vi "Perform Measurement - Single Point.vi"(8 "error in (no error)":errorcluster, 9 "Measure Call Context in":refnum<class "Measure Call Context.lvclass">, 11 "measurement configuration":T2={"Mode of operation"=enum."Power on the DUT", "Source enable/disable"=FALSE, "Load enable/disable"=FALSE, "Power ON/Source resource names"=[], "Load resource names"=[], "Power ON/Source system configuration"=enum."Series", "Power ON/Source output function"=0, "Power ON/Source voltage/current level"=0.0, "Source voltage/current level range"=0.0, "Power ON/Source sense"=0, "Source limit symmetry"=enum."Symmetric", "Power ON/Source current/voltage limit range"=0.0, "Source current/voltage limit low"=0.0, "Source current/voltage limit high"=0.0, "Source transient response"=0, "Source voltage gain bandwidth"=0.0, "Source voltage compensation frequency"=0.0, "Load device voltage/current rating"=30.0, "Source voltage pole-zero ratio"=0.0, "Load system configuration"=enum."Series", "Load output function"=0, "Load voltage/current level"=0.0, "Load voltage/current level range"=0.0, "Load sense"=0, "Load limit symmetry"=enum."Symmetric", "Load current/voltage limit range"=0.0, "Load current/voltage limit low"=0.0, "Load current/voltage limit high"=0.0, "Load transient response"=0, "Load current gain bandwidth"=0.0, "Load current compensation frequency"=0.0, "Load current pole-zero ratio"=0.0, "Aperture time"=0.0, "Measurement duration"=0.0, "Measurement timeout"=1.0} {"Measurement timeout" format="%.3p"; "Load device voltage/current rating" format="%#_6pA"; "Load current compensation frequency" format="%#_6p"; "Load output function" items=["DC Voltage"=1006, "DC Current"=1007, "Pulse Voltage"=1049, "Pulse Current"=1050]; "Power ON/Source output function" items=["DC Voltage"=1006, "DC Current"=1007, "Pulse Voltage"=1049, "Pulse Current"=1050]; "Load sense" items=["Local"=1008, "Remote"=1009]; "Load transient response" items=["Slow"=1041, "Normal"=1038, "Fast"=1039, "Custom"=1042]; "Power ON/Source sense" items=["Symmetric", "Asymmetric"]; "Source transient response" items=["Slow"=1041, "Normal"=1038, "Fast"=1039, "Custom"=1042]; "Measurement duration" format="%.3p"; "Load current/voltage limit high" format="%#_6p"; "Load current/voltage limit low" format="%#_6p"; "Load current/voltage limit range" format="%#_6p"; "Load voltage/current level range" format="%#_6p"; "Load voltage/current level" format="%#_6p"; "Source current/voltage limit high" format="%#_6p"; "Source current/voltage limit low" format="%#_6p"; "Power ON/Source current/voltage limit range" format="%#_6p"; "Source voltage/current level range" format="%#_6p"; "Power ON/Source voltage/current level" format="%#_6p"}) -> (0 "error out":errorcluster, 1 "Measure Call Context out":refnum<class "Measure Call Context.lvclass">, 3 "Measurement Results":T1)   [LabVIEW 2021, in "Single Point_Channel Ganging.lvlib"]
doc: "This VI Perform different API calls to do Single-Point Measurement in different configurations of Source and Load like \n\nSingle-Ganged \nGanged-Ganged\nGanged-Single\nSingle-Single"
uses:
  Single Point_Channel Ganging.lvlib
  Measurement Configuration.ctl
  Measurement Results.ctl
  <vilib>/Plug-In SDKs/Measurements/Measure Call Context/Measure Call Context.lvclass
  Controls/Perform measurement-control.ctl
  shared subVIs/ctl/NIDCPower_channel_ganging - ctl - ganged session.ctl
  shared subVIs/ctl/NIDCPower_channel_ganging - ctl - ganged config.ctl
  shared subVIs/ctl/NIDCPower_channel_ganging - ctl - channel mode.ctl
  <instrlib>/niDCPower/nidcpower.llb/niDCPower Wait For Event - Event.ctl
  shared/Common/controls/Start and Wait for Event.ctl
  shared/Ganging/controls/Abort Single Point-Ganging.ctl
  shared/Single/controls/Abort Single Point-Single.ctl
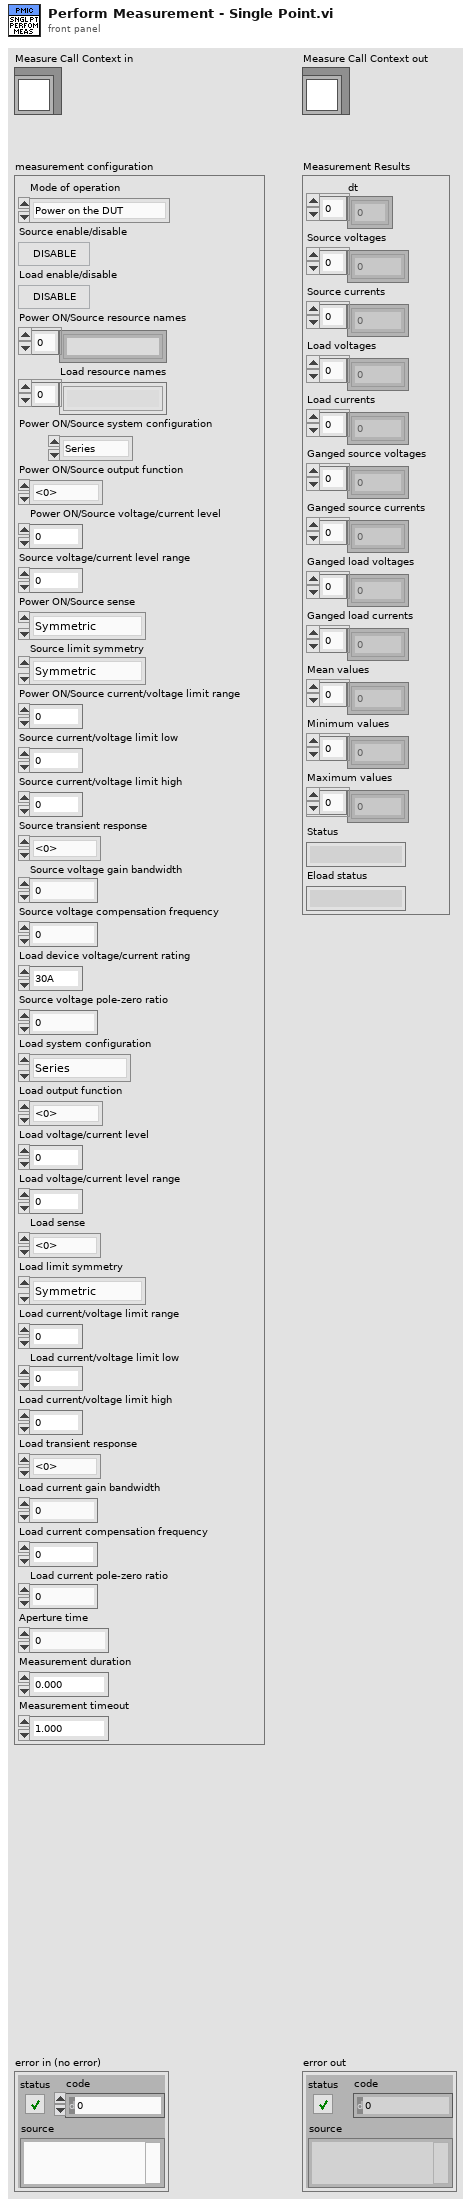
[diagram p1: front panel]
types:
  T1 = typedef "Single Point_Channel Ganging.lvlib/Measurement Results.ctl" = cluster{"dt":dbl[], "Source voltages":dbl[], "Source currents":dbl[], "Load voltages":dbl[], "Load currents":dbl[], "Ganged source voltages":dbl[], "Ganged source currents":dbl[], "Ganged load voltages":dbl[], "Ganged load currents":dbl[], "Mean values":dbl[], "Minimum values":dbl[], "Maximum values":dbl[], "Status":string, "Eload status":string}
  T2 = typedef "Single Point_Channel Ganging.lvlib/Measurement Configuration.ctl" = cluster{"Mode of operation":enum32{"Power on the DUT", "Perform measurement", "Power off the DUT"}, "Source enable/disable":bool, "Load enable/disable":bool, "Power ON/Source resource names":string[], "Load resource names":string[], "Power ON/Source system configuration":enum32{"Series", "Parallel", "Manual"}, "Power ON/Source output function":i32, "Power ON/Source voltage/current level":dbl, "Source voltage/current level range":dbl, "Power ON/Source sense":i32, "Source limit symmetry":enum32{"Symmetric", "Asymmetric"}, "Power ON/Source current/voltage limit range":dbl, "Source current/voltage limit low":dbl, "Source current/voltage limit high":dbl, "Source transient response":i32, "Source voltage gain bandwidth":dbl, "Source voltage compensation frequency":dbl, "Load device voltage/current rating":dbl, "Source voltage pole-zero ratio":dbl, "Load system configuration":enum32{"Series", "Parallel", "Manual"}, "Load output function":i32, "Load voltage/current level":dbl, "Load voltage/current level range":dbl, "Load sense":i32, "Load limit symmetry":enum32{"Symmetric", "Asymmetric"}, "Load current/voltage limit range":dbl, "Load current/voltage limit low":dbl, "Load current/voltage limit high":dbl, "Load transient response":i32, "Load current gain bandwidth":dbl, "Load current compensation frequency":dbl, "Load current pole-zero ratio":dbl, "Aperture time":dbl, "Measurement duration":dbl, "Measurement timeout":dbl}
  T3 = typedef "Single Point_Channel Ganging.lvlib/Perform measurement-control.ctl" = cluster{"Source Ganged Session Out":T4, "Load Ganged Session Out":T4, "Source Measure Record Length":i32, "Load Measure Record Length":i32, "Measurement Results":T1, "Load Slave resource name":string[], "Load Master/Single resource name":string, "Source Slave resource name":string[], "Source Master/Single resource name":string, "Load ganged/single":bool, "Source ganged/single":bool, "Source channel name":string, "Load channel name":string, "Source session out":refnum<k15>, "Load session out":refnum<k15>, "Number of Eload used":i32, "Load Source ON/OFF":enum16{"SOURCE AND LOAD OFF", "SOURCE ON", "LOAD ON", "SOURCE AND LOAD ON"}, "Measurement timeout":dbl}
  T4 = typedef "NIDCPower_channel_ganging - ctl - ganged session.ctl" = cluster{"Ganged Config":T5, "Session List":refnum<k15>[], "Session Mode":T6[], "Channel":string[]}
  T5 = typedef "NIDCPower_channel_ganging - ctl - ganged config.ctl" = enum32{"Series", "Parallel", "Manual"}
  T6 = typedef "NIDCPower_channel_ganging - ctl - channel mode.ctl" = enum32{"Master", "Slave", "Slave - Inverted"}
  T7 = typedef "Start and Wait for Event.ctl" = cluster{"Source Ganged Session Out":T4, "Load Ganged Session Out":T4, "Source session out":refnum<k15>, "Load session out":refnum<k15>, "event":T8, "Source channel name":string, "Load channel name":string, "Load Source ON/OFF":enum16{"SOURCE AND LOAD OFF", "SOURCE ON", "LOAD ON", "SOURCE AND LOAD ON"}, "Load ganged/single":bool, "Source ganged/single":bool}
  T8 = typedef "niDCPower Wait For Event - Event.ctl" = i32
  T9 = typedef "Abort Single Point-Ganging.ctl" = cluster{"Ganged Session in":cluster{"Ganged Config":T5, "Session List":refnum<k15>[], "Session Mode":T6[], "Channel":string[]}}
  T10 = typedef "Abort Single Point-Single.ctl" = cluster{"Resource out":refnum<k15>, "Resource channel name":string}
  T11 = enum32{"Power on the DUT", "Perform measurement", "Power off the DUT"}
  T12 = enum16{"SOURCE AND LOAD OFF", "SOURCE ON", "LOAD ON", "SOURCE AND LOAD ON"}
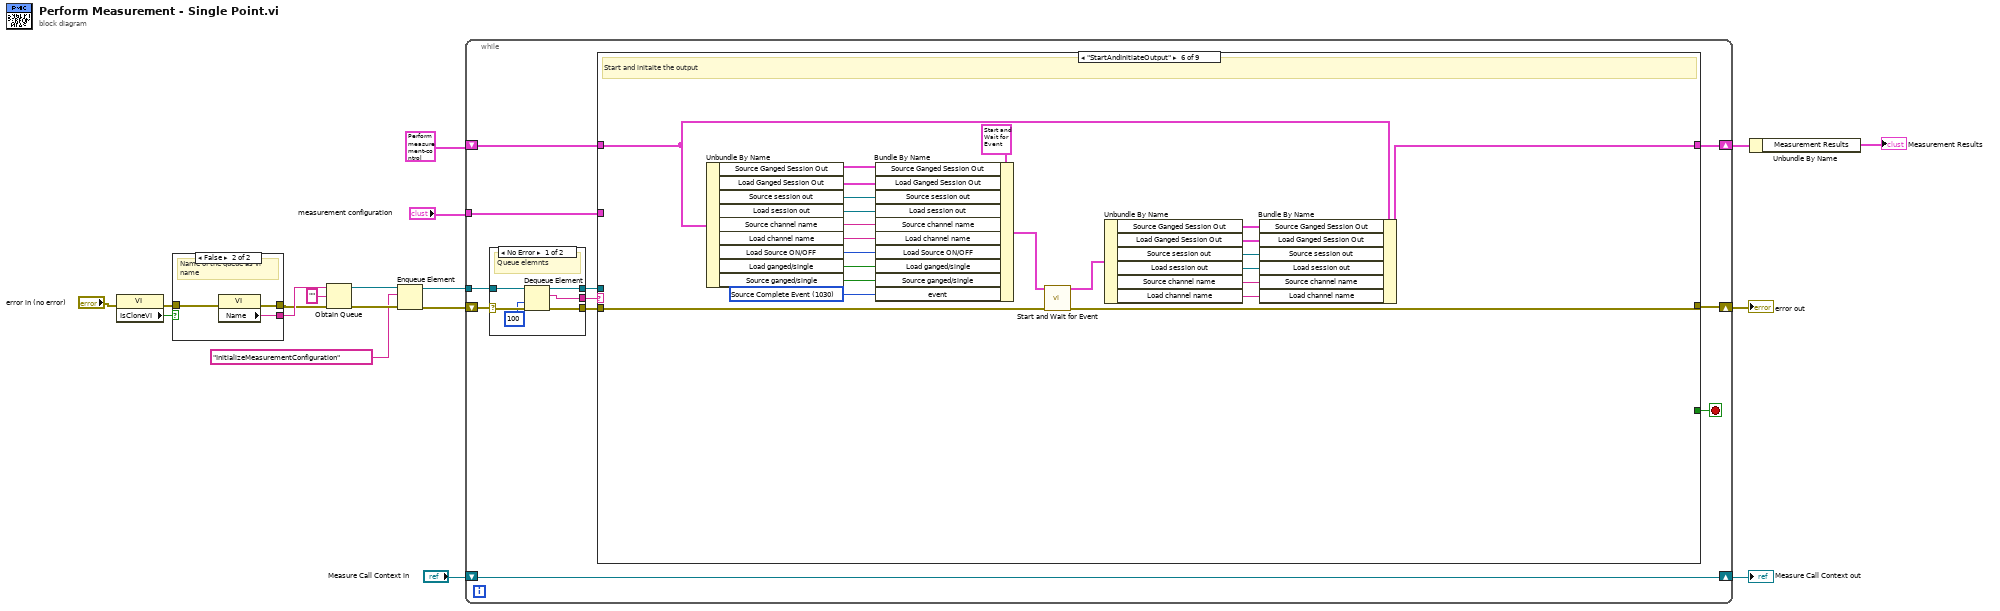
[diagram p0: block diagram]
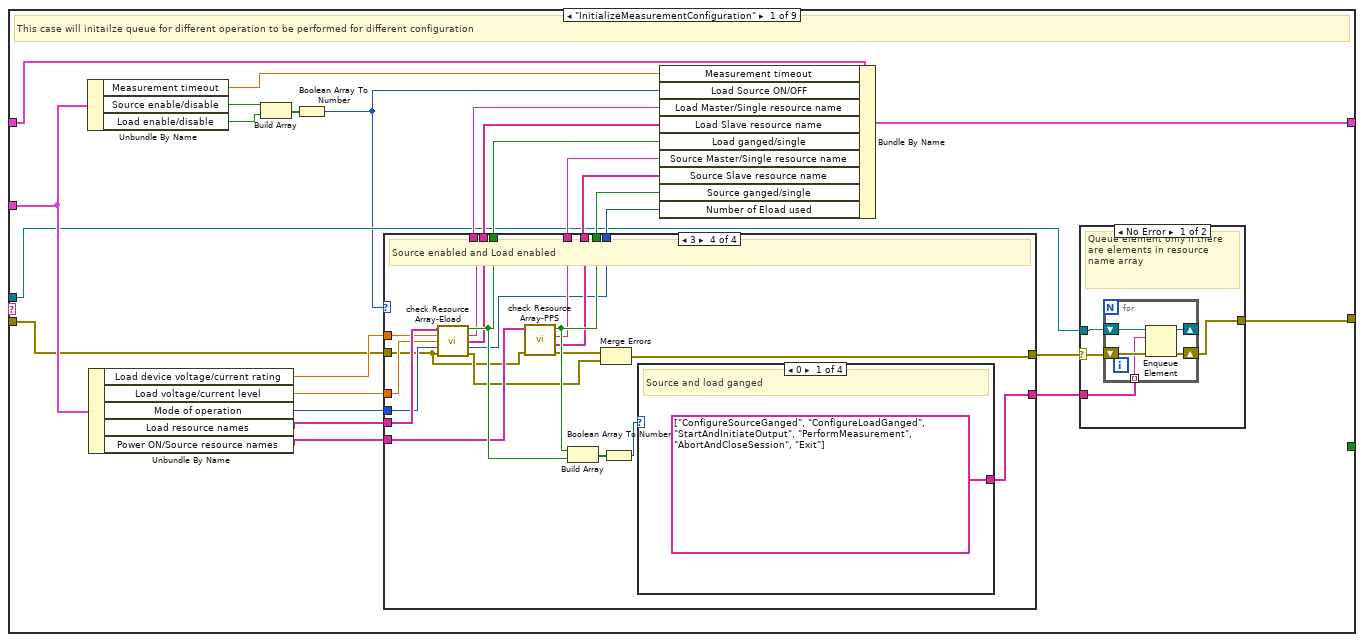
[diagram p2: hidden frame]
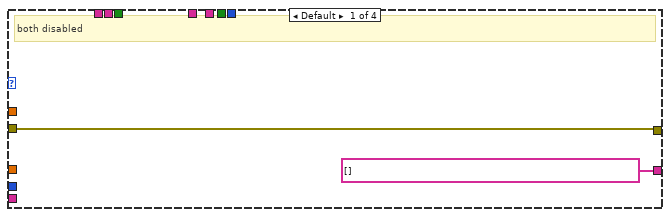
[diagram p4: hidden frame]
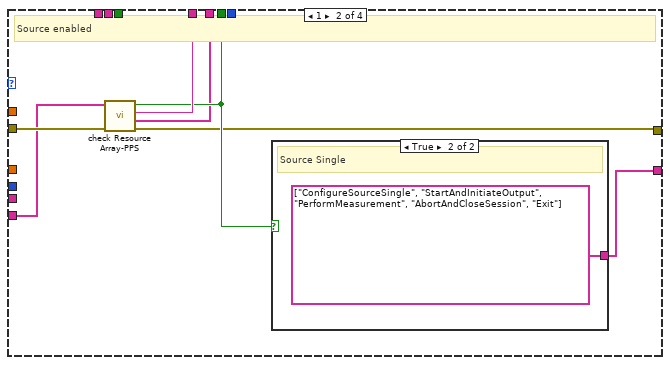
[diagram p5: hidden frame]
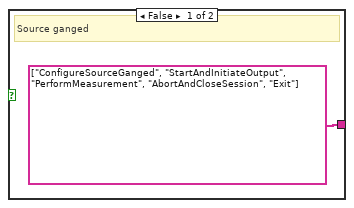
[diagram p6: hidden frame]
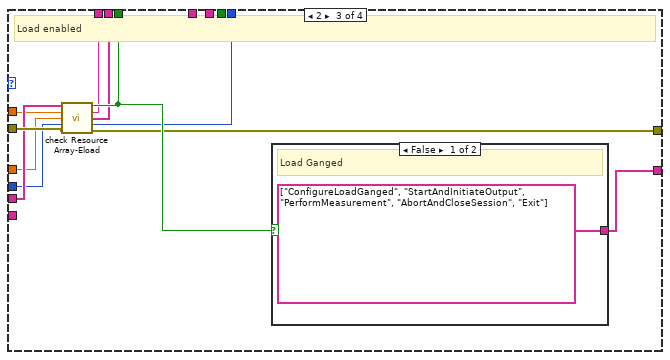
[diagram p7: hidden frame]
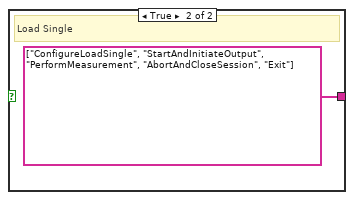
[diagram p8: hidden frame]
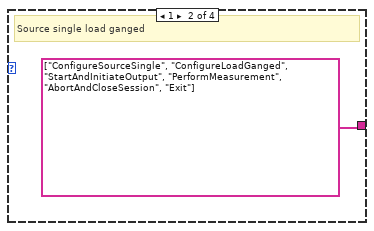
[diagram p9: hidden frame]
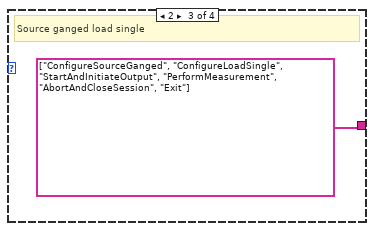
[diagram p10: hidden frame]
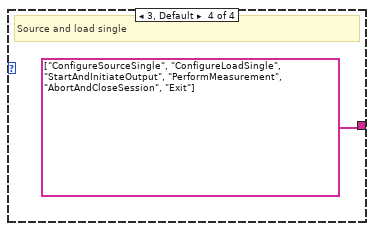
[diagram p11: hidden frame]
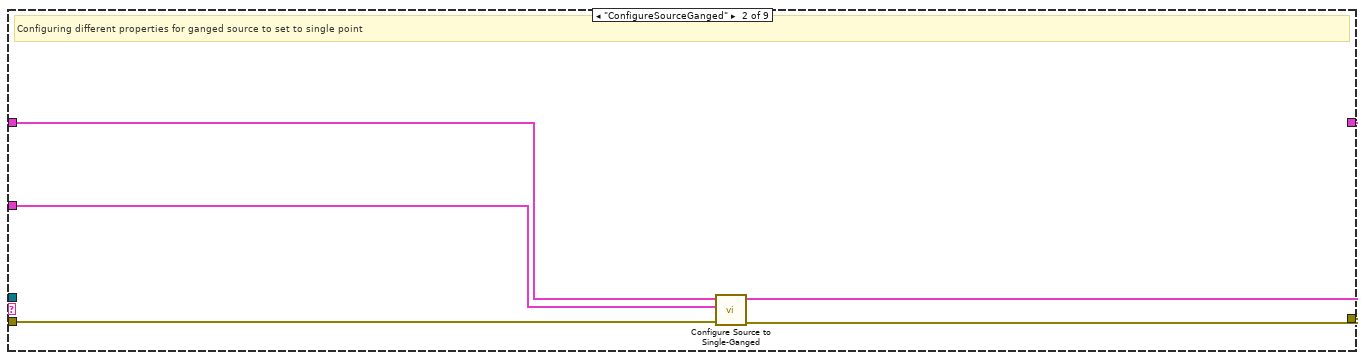
[diagram p12: hidden frame]
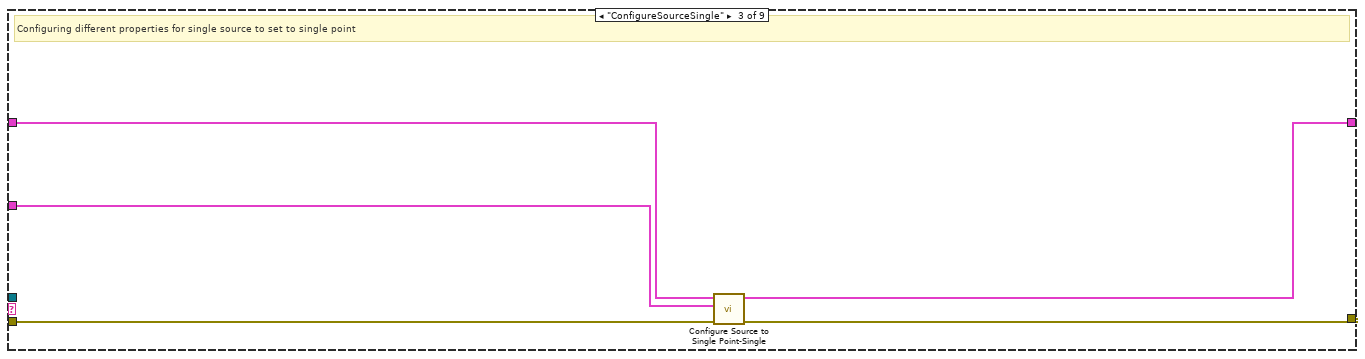
[diagram p13: hidden frame]
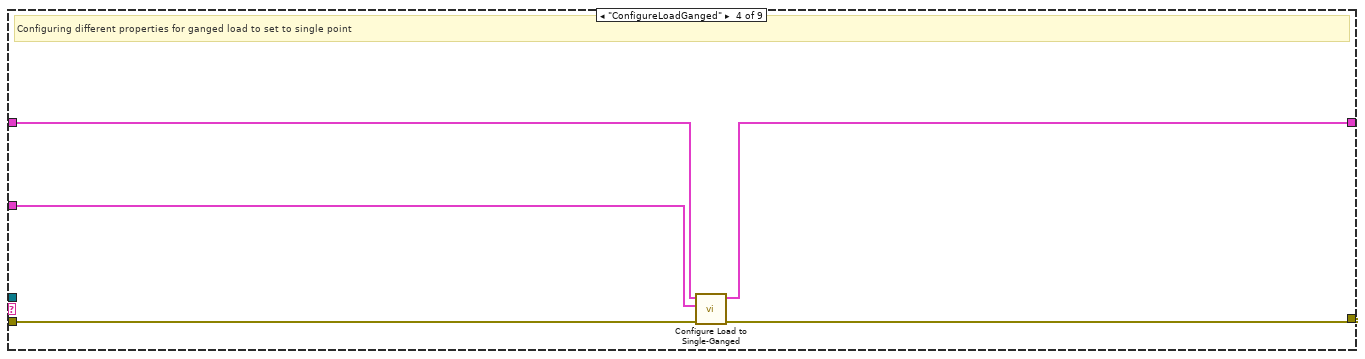
[diagram p14: hidden frame]
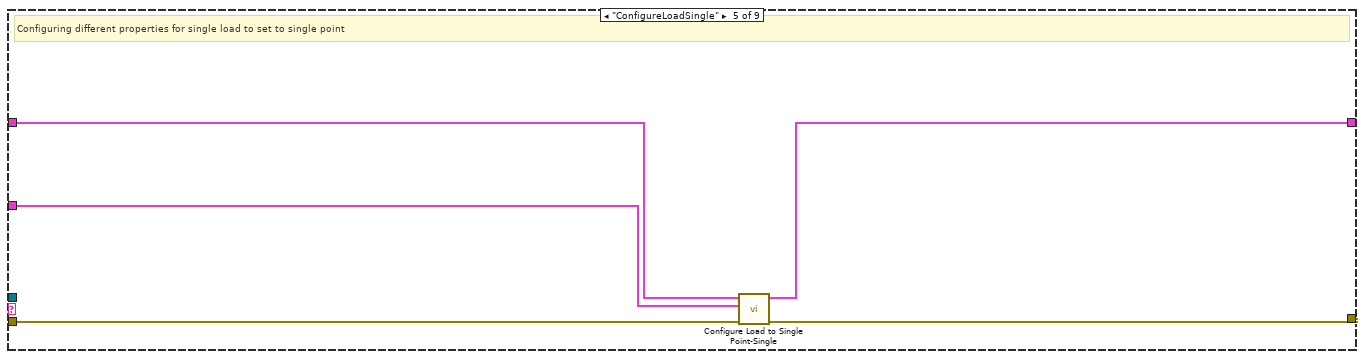
[diagram p15: hidden frame]
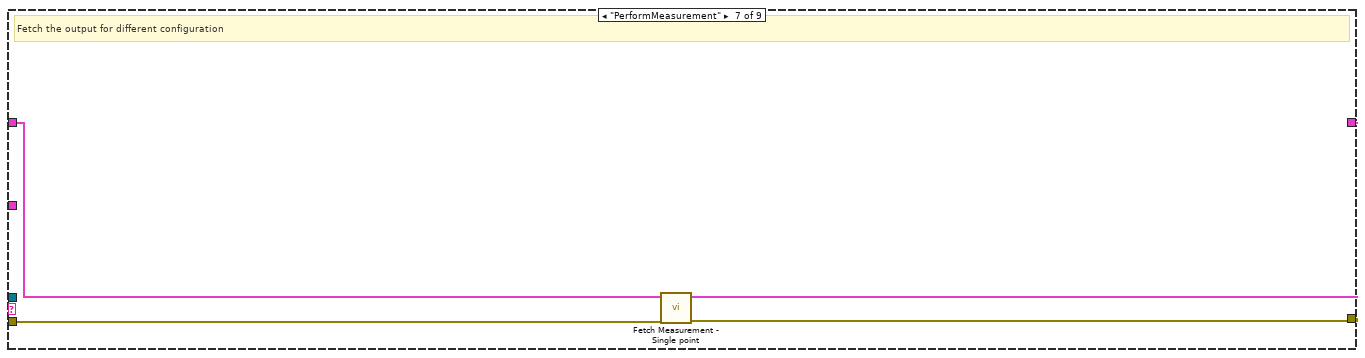
[diagram p16: hidden frame]
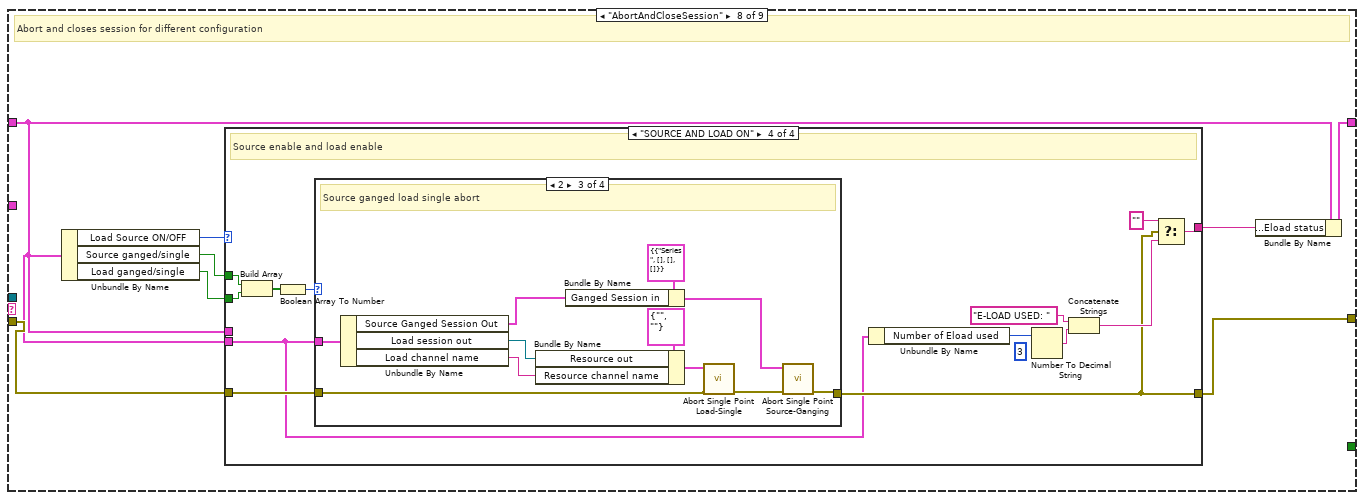
[diagram p17: hidden frame]
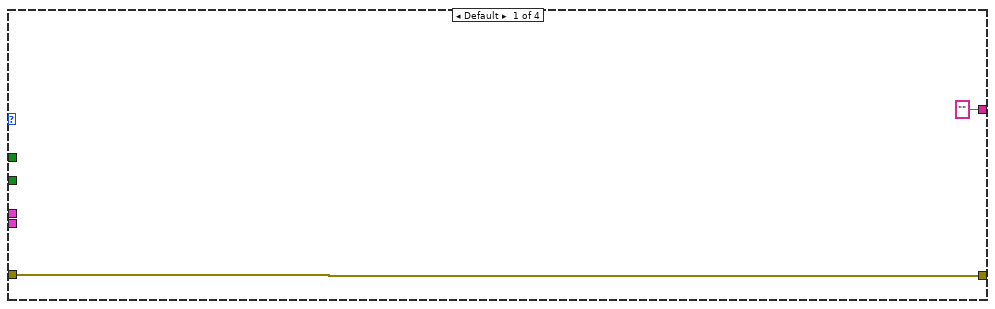
[diagram p18: hidden frame]
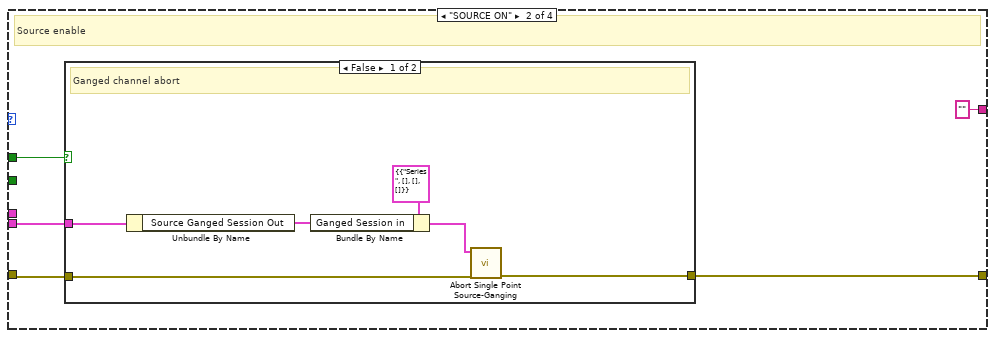
[diagram p19: hidden frame]
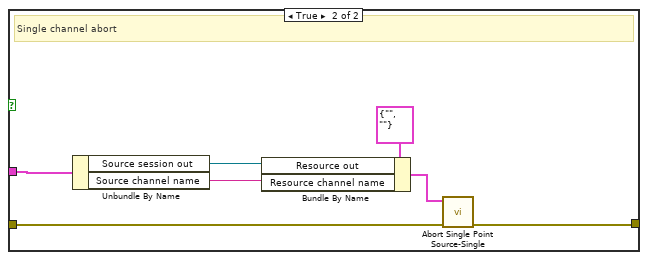
[diagram p20: hidden frame]
diagram:
  n1 = property class="VI"(error in="error in (no error)") -> (error out=w7:errorcluster, "IsCloneVI"=w6:bool)  [unwired: 1 in, 1 out]
  n2 = case shown="False" w6 {
    tunnel: [w21 w24] -> w8
    tunnel: [w20 w23] -> w10
    tunnel: w7 -> [w19 w22]
    frame True {
      # "Name of the queue as vi clone name"
      n3 = property class="VI"(error in=w19) -> (error out=w21:errorcluster, "Clone Name"=w20:string)  [unwired: 1 in, 1 out]
    }
    frame False {
      # "Name of the queue as vi name"
      n4 = property class="VI"(error in=w22) -> (error out=w24:errorcluster, "Name"=w23:string)  [unwired: 1 in, 1 out]
    }
  }
  n5 = Obtain Queue(name (unnamed)=w10, element data type="", error in (no error)=w8) -> (queue out=w4:refnum<queue>, error out=w5:errorcluster)  [unwired: 2 in, 1 out]
  n6 = Enqueue Element(queue=w4, element="InitializeMeasurementConfiguration" ("Step sequence"), error in (no error)=w5) -> (queue out=w11:refnum<queue>, error out=w12:errorcluster)  [unwired: 1 in, 1 out]
  n7 = while {
    tunnel: w11 -> [w35]
    shift-right: [w29] -> w16
    shift-left: T3 {"Source Ganged Session Out"={"Ganged Config"=enum."Series", "Session List"=[], "Session Mode"=[], "Channel"=[]}, "Load Ganged Session Out"={"Ganged Config"=enum."Series", "Session List"=[], "Session Mode"=[], "Channel"=[]}, "Source Measure Record Length"=0, "Load Measure Record Length"=0, "Measurement Results"={"dt"=[], "Source voltages"=[], "Source currents"=[], "Load voltages"=[], "Load currents"=[], "Ganged source voltages"=[], "Ganged source currents"=[], "Ganged load voltages"=[], "Ganged load currents"=[], "Mean values"=[], "Minimum values"=[], "Maximum values"=[], "Status"="", "Eload status"=""}, "Load Slave resource name"=[], "Load Master/Single resource name"="", "Source Slave resource name"=[], "Source Master/Single resource name"="", "Load ganged/single"=FALSE, "Source ganged/single"=FALSE, "Source channel name"="", "Load channel name"="", "Source session out"="", "Load session out"="", "Number of Eload used"=0, "Load Source ON/OFF"=enum."SOURCE AND LOAD ON", "Measurement timeout"=0.0} -> [w30]
    shift-right: [w28] -> w15
    shift-left: w12 -> [w34]
    shift-right: [w27] -> w14
    shift-left: "Measure Call Context in" -> [w27]
    tunnel: "measurement configuration" -> [w25]
    stop <- w26 stop-if-true
    n8 = case shown="No Error" w34 {
      selector: w34 -> [w281 w285]
      tunnel: w35 -> [w283 w284]
      tunnel: [w282 "Exit" ("t")] -> w33
      tunnel: [w280 w285] -> w31
      tunnel: [w278 w284] -> w32
      frame No Error {
        # "Queue elemnts"
        n9 = Dequeue Element(queue=w283, timeout in ms (-1)=100, error in (no error)=w281) -> (queue out=w278:refnum<queue>, element=w282:string, error out=w280:errorcluster)  [unwired: 1 out]
      }
      frame Error {
        # "Go to Exit case"
      }
    }
    n10 = case shown="\"StartAndInitiateOutput\"" w33 {
      tunnel: w32 -> [w40 _ _ _ _ _ _ _ _]
      tunnel: w31 -> [w41 w118 w127 w128 w137 w141 w164 w167 w275]
      tunnel: w30 -> [w45 w119 w123 w130 w135 w138 w161 w166 w276]
      tunnel: [w42 w122 w124 w132 w133 w139 w163 w168 w276] -> w29
      tunnel: [w43 w121 w125 w131 w134 w140 w162 w169 w275] -> w28
      tunnel: [_ _ _ _ _ _ _ _ TRUE] -> w26
      tunnel: w25 -> [w44 w120 w126 w129 w136 _ _ _ _]
      frame "InitializeMeasurementConfiguration" {
        # "This case will initailze queue for different operation to be performed for different configuration"
        n11 = Unbundle By Name(w44) -> ("Measurement timeout"=w38:dbl, "Source enable/disable"=w50:bool, "Load enable/disable"=w49:bool)
        n12 = Unbundle By Name(w44) -> ("Load device voltage/current rating"=w59:dbl, "Load voltage/current level"=w60:dbl, "Mode of operation"=w36:T11, "Load resource names"=w51:string[], "Power ON/Source resource names"=w52:string[])
        n13 = Build Array(w50, w49) -> (w48:bool[])
        n14 = Boolean Array To Number(Boolean array=w48) -> (number=w39:u32)
        n15 = case shown="3" w39 {
          tunnel: w41 -> [w71 w79 w92 w95]
          tunnel: [w71 w74 w86 w99] -> w37
          tunnel: w51 -> [_ _ w91 w111]
          tunnel: w52 -> [_ w78 _ w104]
          tunnel: [_ _ w89 w109] -> w53
          tunnel: [_ _ w88 w108] -> w54
          tunnel: [_ w77 _ w106] -> w55
          tunnel: [_ w75 _ w105] -> w56
          tunnel: [_ _ w90 w110] -> w57
          tunnel: [_ w76 _ w107] -> w58
          tunnel: w59 -> [_ _ w87 w103]
          tunnel: w60 -> [_ _ w83 w97]
          tunnel: [string[] [] ("Step sequence") w73 w85 w100] -> w47
          tunnel: [_ _ w84 w101] -> w46
          tunnel: w36 -> [_ _ w82 w96]
          frame Default {
            # "both disabled"
          }
          frame 1 {
            # "Source enabled"
            n16 = call "check Resource Array-PPS.vi"("error in"=w79, "Resource names"=w78) -> ("error out"=w74:errorcluster, "Slave resource names"=w75:string[], "Single/Master resouce names"=w77:string, "Single or ganged configuration"=w76:bool)  [unwired: 6 in]
            n17 = case shown="True" w76 {
              tunnel: [string[] ["ConfigureSourceGanged", "StartAndInitiateOutput", "PerformMeasurement", "AbortAndCloseSession", "Exit"] ("Step sequence") string[] ["ConfigureSourceSingle", "StartAndInitiateOutput", "PerformMeasurement", "AbortAndCloseSession", "Exit"] ("Step sequence")] -> w73
              frame False {
                # "Source ganged"
              }
              frame True {
                # "Source Single"
              }
            }
          }
          frame 2 {
            # "Load enabled"
            n18 = call "check Resource Array-Eload.vi"("Resource names"=w91, "Device current rating"=w87, "Expected current level"=w83, "Mode of operation"=w82, "error in"=w92) -> ("Single or ganged configuration"=w90:bool, "Single/Master resouce name"=w89:string, "Slave resource names"=w88:string[], "Number of devices used"=w84:i32, "error out"=w86:errorcluster)  [unwired: 6 in]
            n19 = case shown="False" w90 {
              tunnel: [string[] ["ConfigureLoadGanged", "StartAndInitiateOutput", "PerformMeasurement", "AbortAndCloseSession", "Exit"] ("Step sequence") string[] ["ConfigureLoadSingle", "StartAndInitiateOutput", "PerformMeasurement", "AbortAndCloseSession", "Exit"] ("Step sequence")] -> w85
              frame False {
                # "Load Ganged"
              }
              frame True {
                # "Load Single"
              }
            }
          }
          frame 3 {
            # "Source enabled and Load enabled"
            n20 = call "check Resource Array-Eload.vi"("Resource names"=w111, "Device current rating"=w103, "Expected current level"=w97, "Mode of operation"=w96, "error in"=w95) -> ("Single or ganged configuration"=w110:bool, "Single/Master resouce name"=w109:string, "Slave resource names"=w108:string[], "Number of devices used"=w101:i32, "error out"=w98:errorcluster)  [unwired: 6 in]
            n21 = call "check Resource Array-PPS.vi"("error in"=w95, "Resource names"=w104) -> ("error out"=w102:errorcluster, "Slave resource names"=w105:string[], "Single/Master resouce names"=w106:string, "Single or ganged configuration"=w107:bool)  [unwired: 6 in]
            n22 = Build Array(w107, w110) -> (w113:bool[])
            n23 = Merge Errors(w102, w98) -> (w99:errorcluster)
            n24 = Boolean Array To Number(Boolean array=w113) -> (number=w112:u32)
            n25 = case shown="0" w112 {
              tunnel: [string[] ["ConfigureSourceGanged", "ConfigureLoadGanged", "StartAndInitiateOutput", "PerformMeasurement", "AbortAndCloseSession", "Exit"] ("Step sequence") string[] ["ConfigureSourceSingle", "ConfigureLoadGanged", "StartAndInitiateOutput", "PerformMeasurement", "AbortAndCloseSession", "Exit"] ("Step sequence") string[] ["ConfigureSourceGanged", "ConfigureLoadSingle", "StartAndInitiateOutput", "PerformMeasurement", "AbortAndCloseSession", "Exit"] ("Step sequence") string[] ["ConfigureSourceSingle", "ConfigureLoadSingle", "StartAndInitiateOutput", "PerformMeasurement", "AbortAndCloseSession", "Exit"] ("Step sequence")] -> w100
              frame 0 {
                # "Source and load ganged"
              }
              frame 1 {
                # "Source single load ganged"
              }
              frame 2 {
                # "Source ganged load single"
              }
              frame 3, Default {
                # "Source and load single"
              }
            }
          }
        }
        n26 = Bundle By Name(cluster=w45, "Measurement timeout"=w38, "Load Source ON/OFF"=w39, "Load Master/Single resource name"=w53, "Load Slave resource name"=w54, "Load ganged/single"=w57, "Source Master/Single resource name"=w55, "Source Slave resource name"=w56, "Source ganged/single"=w58, "Number of Eload used"=w46) -> (w42:T3)
        n27 = case shown="No Error" w37 {
          selector: w37 -> [w61 w70]
          tunnel: w47 -> [w64 _]
          tunnel: [w63 w70] -> w43
          tunnel: w40 -> [w62 _]
          frame No Error {
            # "Queue element only if there are elements in resource name array"
            n28 = for {
              shift-right: [w67] -> _
              shift-left: w62 -> [w69]
              shift-right: [w66] -> w63
              shift-left: w61 -> [w68]
              tunnel: w64 -> [w65] mode=indexing
              n29 = Enqueue Element(queue=w69, element=w65, error in (no error)=w68) -> (queue out=w67:refnum<queue>, error out=w66:errorcluster)  [unwired: 1 in, 1 out]
            }
          }
          frame Error {
            # "If error directly goes to exit case"
          }
        }
      }
      frame "ConfigureSourceGanged" {
        # "Configuring different properties for ganged source to set to single point"
        n30 = call "Configure Source to Single-Ganged.vi"("error in"=w118, "measurement configuration"=w120, "Single Point Perform Measurement in"=w119) -> ("error out"=w121:errorcluster, "Single Point Perform Measurement out"=w122:T3)  [unwired: 7 in]
      }
      frame "ConfigureSourceSingle" {
        # "Configuring different properties for single source to set to single point"
        n31 = call "Configure Source to Single Point-Single.vi"("error in"=w127, "measurement configuration"=w126, "Single Point Perform Measurement in"=w123) -> ("error out"=w125:errorcluster, "Single Point Perform Measurement out"=w124:T3)  [unwired: 7 in]
      }
      frame "ConfigureLoadGanged" {
        # "Configuring different properties for ganged load to set to single point"
        n32 = call "Configure Load to Single-Ganged.vi"("error in"=w128, "measurement configuration"=w129, "Single Point Perform Measurement in"=w130) -> ("error out"=w131:errorcluster, "Single Point Perform Measurement out"=w132:T3)  [unwired: 7 in]
      }
      frame "ConfigureLoadSingle" {
        # "Configuring different properties for single load to set to single point"
        n33 = call "Configure Load to Single Point-Single.vi"("error in"=w137, "measurement configuration"=w136, "Single Point Perform Measurement in"=w135) -> ("error out"=w134:errorcluster, "Single Point Perform Measurement out"=w133:T3)  [unwired: 7 in]
      }
      frame "StartAndInitiateOutput" {
        w152 = T8 1030 items=["Source Complete Event"=1030, "Measure Complete Event"=1031, "Sequence Iteration Complete Event"=1032, "Sequence Engine Done Event"=1033, "Pulse Complete Event"=1051, "Ready For Pulse Trigger Event"=1052] ("event")
        # "Start and initaite the output"
        n34 = Unbundle By Name(w138) -> ("Source Ganged Session Out"=w160:T4, "Load Ganged Session Out"=w159:T4, "Source session out"=w158:refnum<k15>, "Load session out"=w157:refnum<k15>, "Source channel name"=w156:string, "Load channel name"=w155:string, "Load Source ON/OFF"=w142:T12, "Load ganged/single"=w154:bool, "Source ganged/single"=w153:bool)
        n35 = Bundle By Name(cluster=T7 {"Source Ganged Session Out"={"Ganged Config"=enum."Series", "Session List"=[], "Session Mode"=[], "Channel"=[]}, "Load Ganged Session Out"={"Ganged Config"=enum."Series", "Session List"=[], "Session Mode"=[], "Channel"=[]}, "Source session out"="", "Load session out"="", "event"=1030, "Source channel name"="", "Load channel name"="", "Load Source ON/OFF"=enum."SOURCE ON", "Load ganged/single"=FALSE, "Source ganged/single"=FALSE} ("Start and wait event config"), "Source Ganged Session Out"=w160, "Load Ganged Session Out"=w159, "Source session out"=w158, "Load session out"=w157, "Source channel name"=w156, "Load channel name"=w155, "Load Source ON/OFF"=w142, "Load ganged/single"=w154, "Source ganged/single"=w153, "event"=w152) -> (w143:T7)
        n36 = call "Start and Wait for Event.vi"("error in"=w141, "Start and wait event config"=w143) -> ("error out"=w140:errorcluster, "Start and wait event result"=w145:T7)  [unwired: 7 in]
        n37 = Unbundle By Name(w145) -> ("Source Ganged Session Out"=w151:T4, "Load Ganged Session Out"=w150:T4, "Source session out"=w149:refnum<k15>, "Load session out"=w148:refnum<k15>, "Source channel name"=w147:string, "Load channel name"=w146:string)
        n38 = Bundle By Name(cluster=w138, "Source Ganged Session Out"=w151, "Load Ganged Session Out"=w150, "Source session out"=w149, "Load session out"=w148, "Source channel name"=w147, "Load channel name"=w146) -> (w139:T3)
      }
      frame "PerformMeasurement" {
        # "Fetch the output for different configuration"
        n39 = call "Fetch Measurement - Single point.vi"("error in"=w164, "Single point perform measurement"=w161) -> ("error out"=w162:errorcluster, "Single point perform measurement"=w163:T3)  [unwired: 8 in]
      }
      frame "AbortAndCloseSession" {
        # "Abort and closes session for different configuration"
        n40 = Unbundle By Name(w166) -> ("Load Source ON/OFF"=w172:T12, "Source ganged/single"=w170:bool, "Load ganged/single"=w171:bool)
        n41 = case shown="\"SOURCE AND LOAD ON\"" w172 {
          tunnel: w170 -> [_ w179 _ w229]
          tunnel: w166 -> [_ w178 w203 w218]
          tunnel: w171 -> [_ _ w201 w230]
          tunnel: [w174 w177 w202 w219] -> w169
          tunnel: w167 -> [w174 w176 w204 w226]
          tunnel: w166 -> [_ _ w196 _]
          tunnel: ["" "" w193 w220] -> w165
          frame Default {
          }
          frame "SOURCE ON" {
            # "Source enable"
            n42 = case shown="False" w179 {
              tunnel: w178 -> [w185 w192]
              tunnel: [w182 w187] -> w177
              tunnel: w176 -> [w181 w188]
              frame False {
                # "Ganged channel abort"
                n43 = Unbundle By Name(w185) -> ("Source Ganged Session Out"=w183:T4)
                n44 = Bundle By Name(cluster=T9 {"Ganged Session in"={"Ganged Config"=enum."Series", "Session List"=[], "Session Mode"=[], "Channel"=[]}} ("Ganged Session Out"), "Ganged Session in"=w183) -> (w180:T9)
                n45 = call "Abort Single Point Source-Ganging.vi"("error in"=w181, "Ganged Session In"=w180) -> ("error out"=w182:errorcluster)  [unwired: 9 in]
              }
              frame True {
                # "Single channel abort"
                n46 = Unbundle By Name(w192) -> ("Source session out"=w191:refnum<k15>, "Source channel name"=w190:string)
                n47 = Bundle By Name(cluster=T10 {"Resource out"="", "Resource channel name"=""} ("Abort Single Point - Single"), "Resource out"=w191, "Resource channel name"=w190) -> (w186:T10)
                n48 = call "Abort Single Point Source-Single.vi"("error in"=w188, "Abort Single Point - Single"=w186) -> ("error out"=w187:errorcluster)  [unwired: 9 in]
              }
            }
          }
          frame "LOAD ON" {
            # "Load enable"
            n49 = case shown="False" w201 {
              tunnel: w203 -> [w210 w217]
              tunnel: [w206 w213] -> w202
              tunnel: w204 -> [w207 w212]
              frame False {
                # "Ganged channel abort"
                n50 = Unbundle By Name(w210) -> ("Source Ganged Session Out"=w208:T4)
                n51 = Bundle By Name(cluster=T9 {"Ganged Session in"={"Ganged Config"=enum."Series", "Session List"=[], "Session Mode"=[], "Channel"=[]}} ("Ganged Session Out"), "Ganged Session in"=w208) -> (w205:T9)
                n52 = call "Abort Single Point Load-Ganging.vi"("error in"=w207, "Ganged Session In"=w205) -> ("error out"=w206:errorcluster)  [unwired: 9 in]
              }
              frame True {
                # "Single channel abort"
                n53 = Unbundle By Name(w217) -> ("Load session out"=w216:refnum<k15>, "Load channel name"=w215:string)
                n54 = Bundle By Name(cluster=T10 {"Resource out"="", "Resource channel name"=""} ("Abort Single Point - Single"), "Resource out"=w216, "Resource channel name"=w215) -> (w211:T10)
                n55 = call "Abort Single Point Load-Single.vi"("error in"=w212, "Abort Single Point - Single"=w211) -> ("error out"=w213:errorcluster)  [unwired: 9 in]
              }
            }
            n56 = Unbundle By Name(w196) -> ("Number of Eload used"=w199:i32)
            n57 = Number To Decimal String(number=w199, width (-)=i16 3) -> (decimal integer string=w200:string)
            n58 = Concatenate Strings("E-LOAD USED: ", w200) -> (w195:string)
            n59 = Select(t="", s=w202, f=w195) -> (s? t:f=w193:string)
          }
          frame "SOURCE AND LOAD ON" {
            (unwired) i16 3 ("width (-)")
            # "Source enable and load enable"
            n60 = Build Array(w229, w230) -> (w228:bool[])
            n61 = Boolean Array To Number(Boolean array=w228) -> (number=w227:u32)
            n62 = case shown="2" w227 {
              tunnel: w218 -> [w240 w251 w262 w272]
              tunnel: [w234 w243 w254 w263] -> w219
              tunnel: w226 -> [w232 w245 w256 w267]
              frame 0, Default {
                # "Source and load ganged abort"
                n63 = Unbundle By Name(w240) -> ("Source Ganged Session Out"=w238:T4, "Load Ganged Session Out"=w239:T4)
                n64 = Bundle By Name(cluster=T9 {"Ganged Session in"={"Ganged Config"=enum."Series", "Session List"=[], "Session Mode"=[], "Channel"=[]}} ("Ganged Session In"), "Ganged Session in"=w238) -> (w233:T9)
                n65 = Bundle By Name(cluster=T9 {"Ganged Session in"={"Ganged Config"=enum."Series", "Session List"=[], "Session Mode"=[], "Channel"=[]}} ("Ganged Session In"), "Ganged Session in"=w239) -> (w231:T9)
                n66 = call "Abort Single Point Load-Ganging.vi"("error in"=w232, "Ganged Session In"=w231) -> ("error out"=w235:errorcluster)  [unwired: 9 in]
                n67 = call "Abort Single Point Source-Ganging.vi"("error in"=w235, "Ganged Session In"=w233) -> ("error out"=w234:errorcluster)  [unwired: 9 in]
              }
              frame 1 {
                # "Source single load ganged abort"
                n68 = Unbundle By Name(w251) -> ("Source session out"=w249:refnum<k15>, "Source channel name"=w248:string, "Load Ganged Session Out"=w250:T4)
                n69 = Bundle By Name(cluster=T10 {"Resource out"="", "Resource channel name"=""} ("Abort Single Point - Single"), "Resource out"=w249, "Resource channel name"=w248) -> (w241:T10)
                n70 = Bundle By Name(cluster=T9 {"Ganged Session in"={"Ganged Config"=enum."Series", "Session List"=[], "Session Mode"=[], "Channel"=[]}} ("Ganged Session In"), "Ganged Session in"=w250) -> (w242:T9)
                n71 = call "Abort Single Point Load-Ganging.vi"("error in"=w245, "Ganged Session In"=w242) -> ("error out"=w244:errorcluster)  [unwired: 9 in]
                n72 = call "Abort Single Point Source-Single.vi"("error in"=w244, "Abort Single Point - Single"=w241) -> ("error out"=w243:errorcluster)  [unwired: 9 in]
              }
              frame 2 {
                # "Source ganged load single abort"
                n73 = Unbundle By Name(w262) -> ("Source Ganged Session Out"=w259:T4, "Load session out"=w261:refnum<k15>, "Load channel name"=w260:string)
                n74 = Bundle By Name(cluster=T10 {"Resource out"="", "Resource channel name"=""} ("Abort Single Point - Single"), "Resource out"=w261, "Resource channel name"=w260) -> (w252:T10)
                n75 = Bundle By Name(cluster=T9 {"Ganged Session in"={"Ganged Config"=enum."Series", "Session List"=[], "Session Mode"=[], "Channel"=[]}} ("Ganged Session In"), "Ganged Session in"=w259) -> (w253:T9)
                n76 = call "Abort Single Point Load-Single.vi"("error in"=w256, "Abort Single Point - Single"=w252) -> ("error out"=w255:errorcluster)  [unwired: 9 in]
                n77 = call "Abort Single Point Source-Ganging.vi"("error in"=w255, "Ganged Session In"=w253) -> ("error out"=w254:errorcluster)  [unwired: 9 in]
              }
              frame 3 {
                # "Source and load single abort"
                n78 = Unbundle By Name(w272) -> ("Source session out"=w270:refnum<k15>, "Source channel name"=w271:string, "Load session out"=w274:refnum<k15>, "Load channel name"=w273:string)
                n79 = Bundle By Name(cluster=T10 {"Resource out"="", "Resource channel name"=""} ("Abort Single Point - Single"), "Resource out"=w270, "Resource channel name"=w271) -> (w264:T10)
                n80 = Bundle By Name(cluster=T10 {"Resource out"="", "Resource channel name"=""} ("Abort Single Point - Single"), "Resource out"=w274, "Resource channel name"=w273) -> (w266:T10)
                n81 = call "Abort Single Point Load-Single.vi"("error in"=w267, "Abort Single Point - Single"=w266) -> ("error out"=w265:errorcluster)  [unwired: 9 in]
                n82 = call "Abort Single Point Source-Single.vi"("error in"=w265, "Abort Single Point - Single"=w264) -> ("error out"=w263:errorcluster)  [unwired: 9 in]
              }
            }
            n83 = Unbundle By Name(w218) -> ("Number of Eload used"=w224:i32)
            n84 = Number To Decimal String(number=w224) -> (decimal integer string=w225:string)  [unwired: 1 in]
            n85 = Concatenate Strings("E-LOAD USED: ", w225) -> (w222:string)
            n86 = Select(t="", s=w219, f=w222) -> (s? t:f=w220:string)
          }
        }
        n87 = Bundle By Name(cluster=w166, "Measurement Results.Eload status"=w165) -> (w168:T3)
      }
      frame "Exit", Default {
        # "Stops the while loop"
      }
    }
  }
  "error out" <- w15
  "Measure Call Context out" <- w14
  n88 = Unbundle By Name(w16) -> ("Measurement Results"=→"Measurement Results":T1)
